vi "Enqueue data.vi"(0 "Logging queue metadata shift in":T1={"Imaging Protocol"=enum."Live Imaging", "Number of Trials"=0, "Frame Size"=512, "# Averaged frames"=0, "Dwell time (us)"=0.0, "Index of Z-plane"=0, "Timelapse?"=FALSE, "Logging process is active"=FALSE, "Speed logging enabled"=FALSE, "tdms file ref"=refnum, "path"=path "", "Trial Number"=0, "Expected # points acquired"=FALSE, "Manually stopped"=FALSE, "Last trial"=FALSE, "Ch0 data"=[], "Ch1 data"=[], "Ref Data"=[], "Ref Frame Time"=[], "Image Time"=[], "Ref X Length"=0, "Ref Y Length"=0, "# Ref Averaged frames"=0, "Ref Dwell time (us)"=0.0, "Points acquired"={"Ch0 last trial"=0, "Ch1 last trial"=0, "All trials"=0}, "HW Timings File"=refnum} {"Ref Dwell time (us)" format="%#.6g"; "Frame Size" items=["100X100"=100, "128X128"=128, "200X200"=200, "256X256"=256, "512X512"=512, "1024x1024"=1024, "2048x2048"=2048]; "Dwell time (us)" format="%#.6g"}, 1 "Logging queue in":T5, 5 "Chunk of data":T6={"Ch0 data"=[0], "Ch1 data"=[0], "Ref data"=[0], "Ref time data"=[], "Image time data"=[]}, 11 "Error in":errorcluster, 12 "Expected # points acquired":bool, 14 "Manually stopped":bool) -> (3 "Logging queue out":T5, 4 "Logging queue metadata shift out":T1={"Imaging Protocol"=enum."Live Imaging", "Number of Trials"=0, "Frame Size"=512, "# Averaged frames"=0, "Dwell time (us)"=0.0, "Index of Z-plane"=0, "Timelapse?"=FALSE, "Logging process is active"=FALSE, "Speed logging enabled"=FALSE, "tdms file ref"=refnum, "path"=path "", "Trial Number"=0, "Expected # points acquired"=FALSE, "Manually stopped"=FALSE, "Last trial"=FALSE, "Ch0 data"=[], "Ch1 data"=[], "Ref Data"=[], "Ref Frame Time"=[], "Image Time"=[], "Ref X Length"=0, "Ref Y Length"=0, "# Ref Averaged frames"=0, "Ref Dwell time (us)"=0.0, "Points acquired"={"Ch0 last trial"=0, "Ch1 last trial"=0, "All trials"=0}, "HW Timings File"=refnum} {"Ref Dwell time (us)" format="%#.6g"; "Frame Size" items=["100X100"=100, "128X128"=128, "200X200"=200, "256X256"=256, "512X512"=512, "1024x1024"=1024, "2048x2048"=2048]; "Dwell time (us)" format="%#.6g"}, 15 "error out":errorcluster)   [LabVIEW 2017]
uses:
  Typedefs/Logging queue element.ctl
  Typedefs/Imaging Protocols enum.ctl
  Typedefs/Frame Size.ctl
  Typedefs/Acquired points count.ctl
  Typedefs/Data arrays cluster.ctl
  Typedefs/Data queue ref.ctl
panel:
  out "# points queued":i32
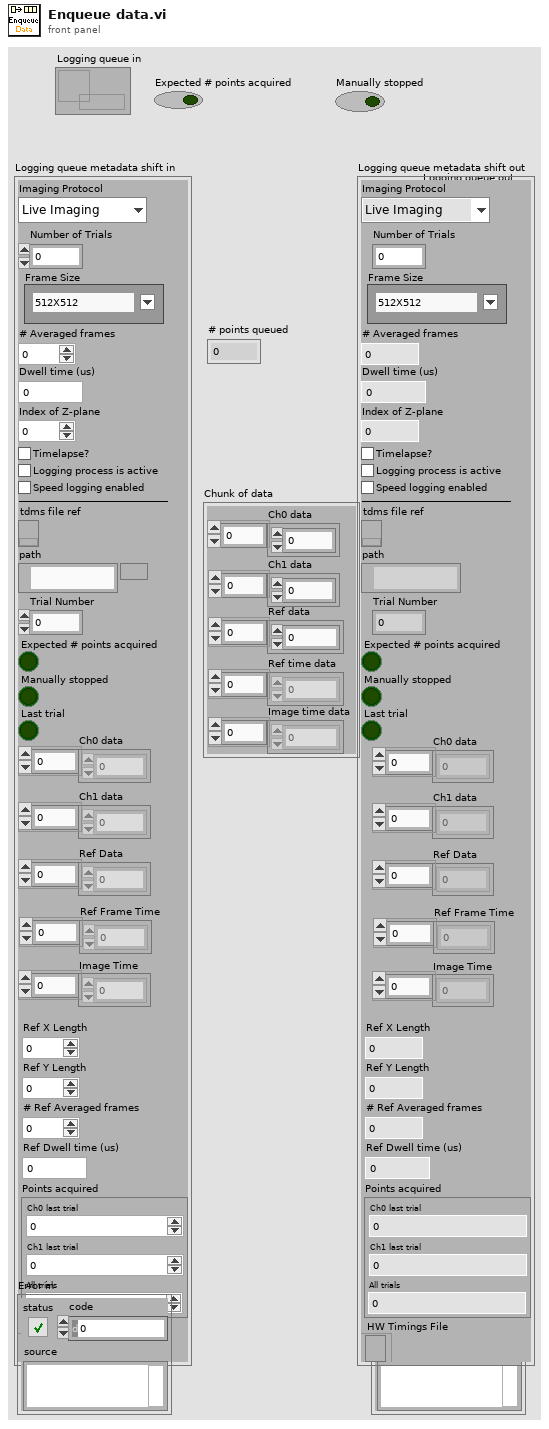
[diagram p1: front panel]
types:
  T1 = typedef "Logging queue element.ctl" = cluster{"Imaging Protocol":T2, "Number of Trials":u16, "Frame Size":T3, "# Averaged frames":u16, "Dwell time (us)":dbl, "Index of Z-plane":i32, "Timelapse?":bool, "Logging process is active":bool, "Speed logging enabled":bool, "tdms file ref":refnum<k34>, "path":path, "Trial Number":i32, "Expected # points acquired":bool, "Manually stopped":bool, "Last trial":bool, "Ch0 data":u32[], "Ch1 data":u32[], "Ref Data":u32[], "Ref Frame Time":u64[], "Image Time":u64[], "Ref X Length":u16, "Ref Y Length":u16, "# Ref Averaged frames":u16, "Ref Dwell time (us)":dbl, "Points acquired":T4, "HW Timings File":refnum<file>}
  T2 = typedef "Imaging Protocols enum.ctl" = enum16{"AOL Z-Stack", "Motor Z Stack", "Functional Acquisition", "Single Plane Acquisition", "Volume Acquisition", "Live Imaging", "Live Plane Imaging", "Live Volume Imaging"}
  T3 = typedef "Frame Size.ctl" = u16
  T4 = typedef "Acquired points count.ctl" = cluster{"Ch0 last trial":u64, "Ch1 last trial":u64, "All trials":u64}
  T5 = typedef "Data queue ref.ctl" = refnum<queue>
  T6 = typedef "Data arrays cluster.ctl" = cluster{"Ch0 data":u32[], "Ch1 data":u32[], "Ref data":u32[], "Ref time data":u64[], "Image time data":u64[]}
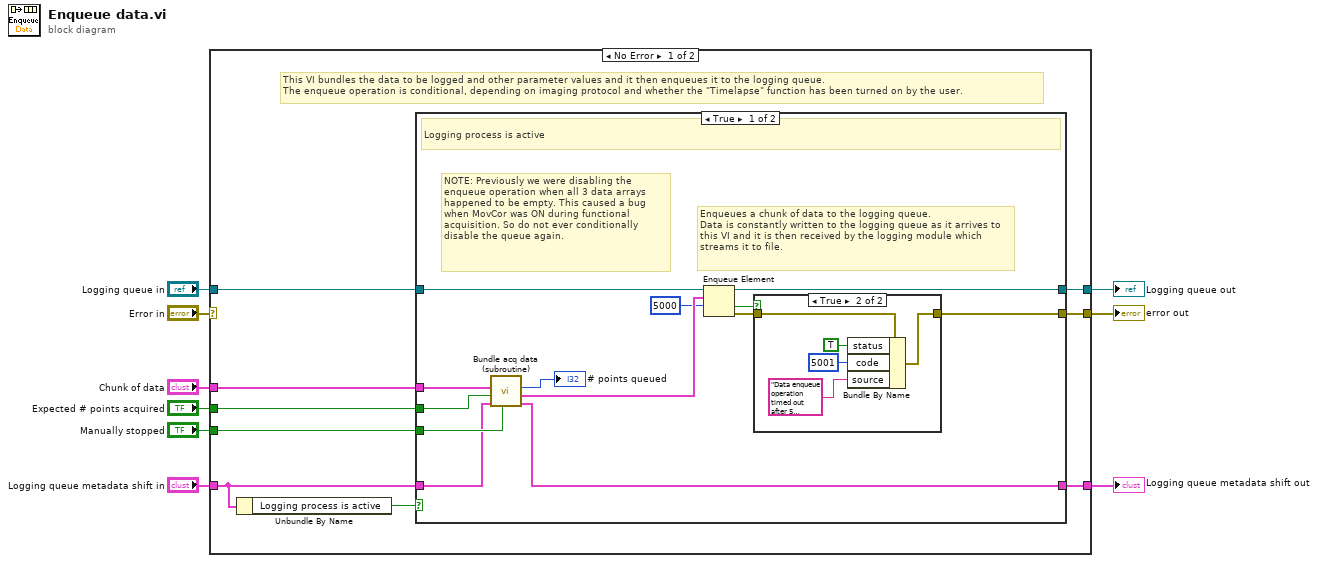
[diagram p0: block diagram]
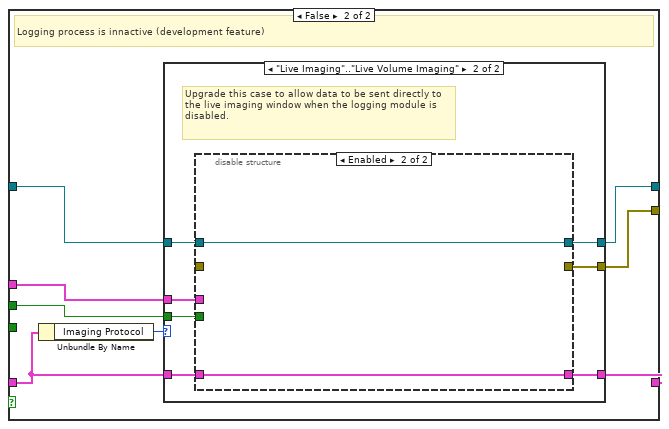
[diagram p3: hidden frame]
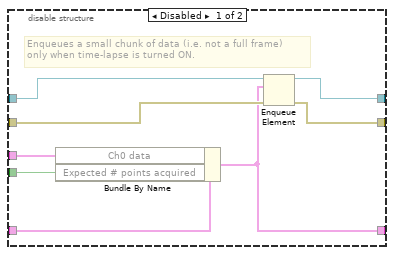
[diagram p5: hidden frame]
diagram:
  n1 = case shown="No Error" "Error in" {
    selector: "Error in" -> [_ w67]
    tunnel: [w17 w67] -> w9
    tunnel: [w16 w66] -> w8
    tunnel: "Logging queue in" -> [w15 w66]
    tunnel: "Chunk of data" -> [w14 _]
    tunnel: [w13 w65] -> w5
    tunnel: "Logging queue metadata shift in" -> [w12 w65]
    tunnel: "Expected # points acquired" -> [w11 _]
    tunnel: "Manually stopped" -> [w10 _]
    frame No Error {
      # "This VI bundles the data to be logged and other parameter values and it then enqueues it to the logging queue.\nThe enqueue operation is conditional, depending on imaging protocol and whether the \"Timelapse\" function has been turned on by the user."
      n2 = Unbundle By Name(w12) -> ("Logging process is active"=w18:bool)
      n3 = case shown="True" w18 {
        tunnel: w12 -> [w25 w40]
        tunnel: w15 -> [w31 w45]
        tunnel: [w30 w44] -> w16
        tunnel: [w29 w43] -> w17
        tunnel: w14 -> [w28 w41]
        tunnel: [w22 w39] -> w13
        tunnel: w11 -> [w27 w38]
        tunnel: w10 -> [w26 _]
        frame True {
          # "NOTE: Previously we were disabling the enqueue operation when all 3 data arrays happened to be empty. This caused a bug when MovCor was ON during functional acquisition. So do not ever conditionally disable the queue again."
          # "Enqueues a chunk of data to the logging queue.\nData is constantly written to the logging queue as it arrives to this VI and it is then received by the logging module which streams it to file."
          # "Logging process is active"
          n4 = call "Bundle acq data (subroutine).vi"("Manually stopped"=w26, "Logging queue metadata shift in"=w25, "Expected # points acquired"=w27, "Chunk of data"=w28) -> ("Logging queue metadata shift out (data removed)"=w22:T1, "Element to queue"=w23:T1, "# points queued"=→"# points queued":i32)  [unwired: 5 in]
          n5 = Enqueue Element(queue=w31, element=w23, timeout in ms (-1)=5000) -> (queue out=w30:T5, timed out?=w19:bool, error out=w20:errorcluster)  [unwired: 1 in]
          n6 = case shown="True" w19 {
            tunnel: w20 -> [w32 w37]
            tunnel: [w32 w36] -> w29
            frame False {
            }
            frame True {
              n7 = Bundle By Name(cluster=w37, "status"=TRUE, "code"=5001, "source"="Data enqueue operation timed out after 5 seconds.") -> (w36:errorcluster)
            }
          }
        }
        frame False {
          # "Logging process is innactive (development feature)"
          n8 = Unbundle By Name(w40) -> ("Imaging Protocol"=w42:T2)
          n9 = case shown="\"Live Imaging\"..\"Live Volume Imaging\"" w42 {
            tunnel: w40 -> [w46 w53]
            tunnel: w45 -> [w47 w49]
            tunnel: [w47 w48] -> w44
            tunnel: [_ w54] -> w43
            tunnel: w41 -> [_ w51]
            tunnel: [w46 w52] -> w39
            tunnel: w38 -> [_ w50]
            frame Default {
            }
            frame "Live Imaging".."Live Volume Imaging" {
              # "Upgrade this case to allow data to be sent directly to the live imaging window when the logging module is disabled."
              n10 = disable-structure shown="Enabled" {
                disable-tunnel: [w62 _] -> w54
                disable-tunnel: _ -> [w61 _]
                disable-tunnel: w53 -> [w60 w63]
                disable-tunnel: [w59 w63] -> w52
                disable-tunnel: w51 -> [w58 _]
                disable-tunnel: w50 -> [w57 _]
                disable-tunnel: w49 -> [w56 w64]
                disable-tunnel: [w55 w64] -> w48
                frame Disabled {
                  # "Enqueues a small chunk of data (i.e. not a full frame)\nonly when time-lapse is turned ON."
                  n11 = Bundle By Name(cluster=w60, "Ch0 data"=w58, "Expected # points acquired"=w57) -> (w59:T1)
                  n12 = Enqueue Element(queue=w56, element=w59, error in (no error)=w61) -> (queue out=w55:T5, error out=w62:errorcluster)  [unwired: 1 in, 1 out]
                }
                frame Enabled {
                }
              }
            }
          }
        }
      }
    }
    frame Error {
    }
  }
  "error out" <- w9
  "Logging queue out" <- w8
  "Logging queue metadata shift out" <- w5
